vi "loadHWConfigurations.vi"(8 "error in (no error)":errorcluster, 11 "StaticOutputEditor in":refnum<class "StaticOutputEditor.lvclass">) -> (0 "error out":errorcluster, 3 "StaticOutputEditor out":refnum<class "StaticOutputEditor.lvclass">)   [LabVIEW 2011, in "Views.lvlib" / "ScriptEditor.lvlib" / "StaticOutputEditor.lvclass"]
uses:
  StaticOutputEditor.lvclass
  StaticOutputEditor.lvclass/StaticOutputEditor.ctl
  Tools/DatabaseHelpers/Database Objects/HWConfiguration/HWConfigurations.lvclass
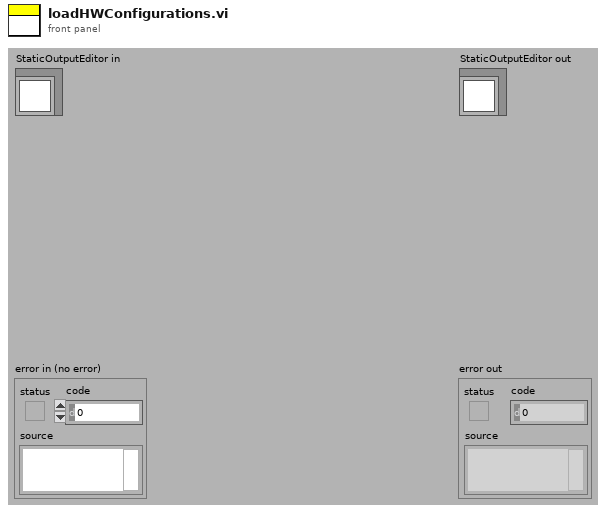
[diagram p1: front panel]
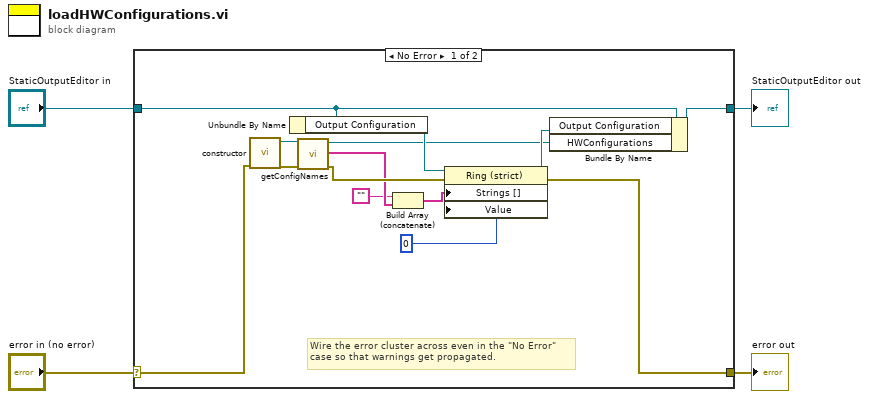
[diagram p0: block diagram]
diagram:
  n1 = case shown="No Error" "error in (no error)" {
    selector: "error in (no error)" -> [w16 w20]
    tunnel: [w5 w20] -> w3
    tunnel: [w7 w19] -> w1
    tunnel: "StaticOutputEditor in" -> [w8 w19]
    frame No Error {
      # "Wire the error cluster across even in the \"No Error\"\ncase so that warnings get propagated."
      n2 = call "constructor.vi"("error in (no error)"=w16) -> ("error out"=w17:errorcluster, "HWConfiguration out"=w18:refnum<class "HWConfigurations.lvclass">)  [unwired: 9 in]
      n3 = Unbundle By Name(w8) -> ("Output Configuration"=w14:refnum<vi>)
      n4 = call "getConfigNames.vi"("error in (no error)"=w17, "HWConfiguration in"=w18) -> ("error out"=w15:errorcluster, "config_names"=w13:string[], "HWConfiguration out"=w6:refnum<class "HWConfigurations.lvclass">)  [unwired: 7 in]
      n5 = Build Array (concatenate)("", w13) -> (w11:string[])
      n6 = property class="Ring (strict)"(reference=w14, error in=w15, "Strings []"=w11, "Value"=0) -> (reference out=w9:refnum<vi>, error out=w5:errorcluster)
      n7 = Bundle By Name(cluster=w8, "Output Configuration"=w9, "HWConfigurations"=w6) -> (w7:refnum<class "StaticOutputEditor.lvclass">)
    }
    frame Error {
    }
  }
  "error out" <- w3
  "StaticOutputEditor out" <- w1
